vi "listbox icon.vi"() -> ()   [LabVIEW 2009]
panel:
  in  "Listbox":i32(listbox)
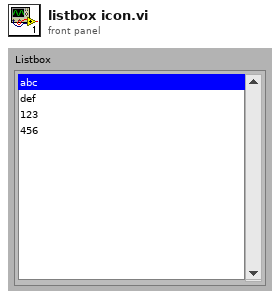
[diagram p1: front panel]
types:
  T1 = typedef "imagedata.ctl" = cluster{"image type":i32, "image depth":i32, "image":u8[], "mask":u8[], "colors":u32[], "Rectangle":cluster{"left":i16, "top":i16, "right":i16, "bottom":i16}}
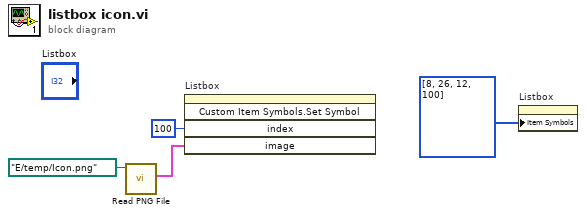
[diagram p0: block diagram]
diagram:
  n1 = call <vilib>:"Read PNG File.vi"("path to PNG file"=path "E:/temp/Icon.png") -> ("image data"=w1:T1)  [unwired: 8 in, 2 out]
  n2 = invoke on="Listbox" class="LstBox (strict)" method="Custom Item Symbols.Set Symbol"("index"=100 ("Index"), "image"=w1) -> ()  [unwired: 3 in, 5 out]
  n3 = property on="Listbox" class="LstBox (strict)"("Item Symbols"=i32[] [8, 26, 12, 100]) -> ()  [unwired: 2 in, 2 out]
